vi "Test State String Through Nested Case Structure.vi"(8 "error in (no error)":errorcluster) -> (0 "error out":errorcluster)   [LabVIEW 2020, in "TEST JKI State Machine API.lvlib"]
uses:
  TEST JKI State Machine API.lvlib
  source/JKI State Machine API.lvlib
  <vilib>/addons/_JKI Toolkits/Caraya/classes/Test/Test.lvclass
  <vilib>/addons/_JKI Toolkits/Caraya/classes/Assert/Assert.lvclass
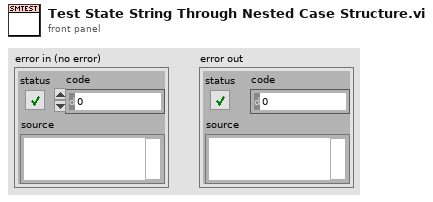
[diagram p1: front panel]
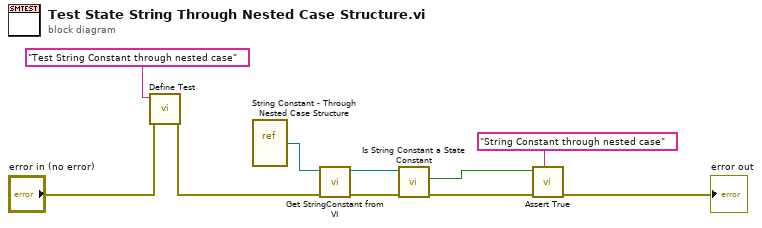
[diagram p0: block diagram]
diagram:
  n1 = call <vilib>:"Define Test.vi"("error in (no error)"="error in (no error)", "Label (VI Title)"="Test String Constant through nested case") -> ("error out"=w9:errorcluster)  [unwired: 8 in, 1 out]
  n2 = vi-ref "String Constant - Through Nested Case Structure.vi"() -> (w6:refnum<vi>)
  n3 = call "Get StringConstant from VI.vi"("error in (no error)"=w9, "VI in"=w6) -> ("error out"=w5:errorcluster, "StringConstant out"=w1:refnum<vi>)  [unwired: 8 in]
  n4 = call "Is String Constant a State Constant.vi"("error in (no error)"=w5, "GObj Refnum"=w1) -> ("error out"=w7:errorcluster, "Is States Constant"=w10:bool)  [unwired: 7 in, 1 out]
  n5 = call <vilib>:"Assert True.vi"("Label"="String Constant through nested case", "error in (no error)"=w7, "True?"=w10) -> ("error out"=→"error out":errorcluster)  [unwired: 7 in, 1 out]
